vi "Shutdown.vi"(8 "error in (no error)":errorcluster, 11 "Log in":refnum<class "Log.lvclass">) -> (0 "error out":errorcluster)   [LabVIEW 2020, in "Log.lvclass"]
doc: "Cleanly shuts down the Log Class, destroying all necessary processes."
uses:
  Log.lvclass
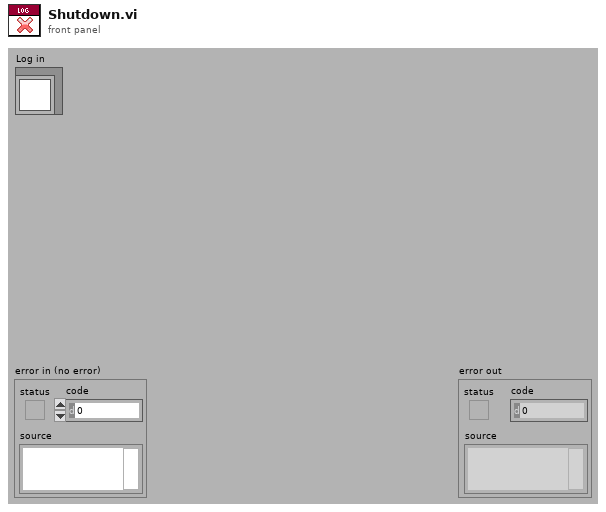
[diagram p1: front panel]
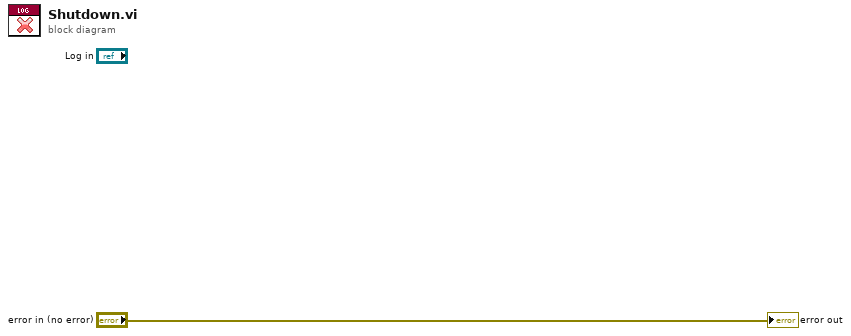
[diagram p0: block diagram]
diagram:
  "error out" <- "error in (no error)"
